vi "Validate Plugin Name.vi"(0 "Project exists?":bool, 5 "Library names":string[](array[string]), 7 "Plug-in name":string, 11 "error in (no error)":errorcluster) -> (4 "Valid Name?":bool, 15 "error out":errorcluster)   [LabVIEW 2021, in "Converter.lvlib"]
uses:
  Converter.lvlib
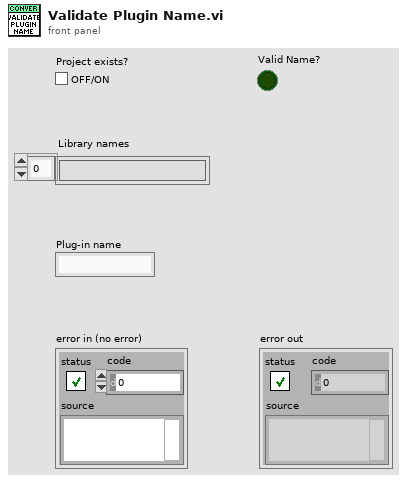
[diagram p1: front panel]
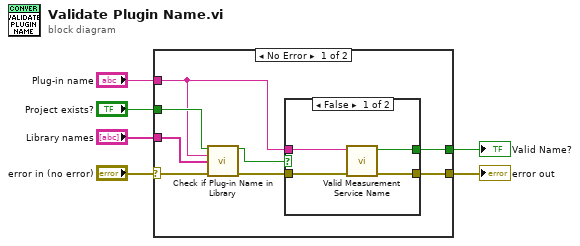
[diagram p0: block diagram]
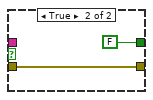
[diagram p2: hidden frame]
diagram:
  n1 = case shown="No Error" "error in (no error)" {
    selector: "error in (no error)" -> [w14 w21]
    tunnel: "Plug-in name" -> [w7 _]
    tunnel: [w13 _] -> w4
    tunnel: [w12 w21] -> w3
    tunnel: "Library names" -> [w8 _]
    tunnel: "Project exists?" -> [w9 _]
    frame No Error {
      n2 = call "Check if Plug-in Name in Library.vi"("Project exists?"=w9, "library name"=w7, "Library names"=w8, "error in (no error)"=w14) -> ("found"=w10:bool, "error out"=w11:errorcluster)  [unwired: 10 in]
      n3 = case shown="False" w10 {
        tunnel: w11 -> [w17 w20]
        tunnel: [w16 FALSE ("valid name?")] -> w13
        tunnel: [w18 w20] -> w12
        tunnel: w7 -> [w15 _]
        frame False {
          n4 = call "Valid Measurement Service Name.vi"("error in"=w17, "requested plugin name"=w15) -> ("error out"=w18:errorcluster, "valid name?"=w16:bool)  [unwired: 8 in]
        }
        frame True {
        }
      }
    }
    frame Error {
    }
  }
  "error out" <- w3
  "Valid Name?" <- w4
